vi "Remove Audio Files from NI ELVIS III.vi"() -> ()   [LabVIEW 2019]
doc: "This VI deletes all the Music files previously uploaded to the target. Only use this VI, after finishing using the Audio Modulation VIs or if you want to transfere other files."
uses:
  <vilib>/FTP/NI_FTP.lvlib
panel:
  in  "Message":string
  out "error out":errorcluster
  in  "error in (no error)":errorcluster
  in  "Host ID":string="172.22.11.2"
  # "Remove Audio Files from NI ELVIS III"
  # "This VI deletes all the Music files previously uploaded to the target. Only use this VI, after finishing using the Audio Modulation VIs or if you want to transfere other files.\n\nRemember that if you want to make use of the Demo once again, you should upload the Audio files once more to the NI ELVIS III."
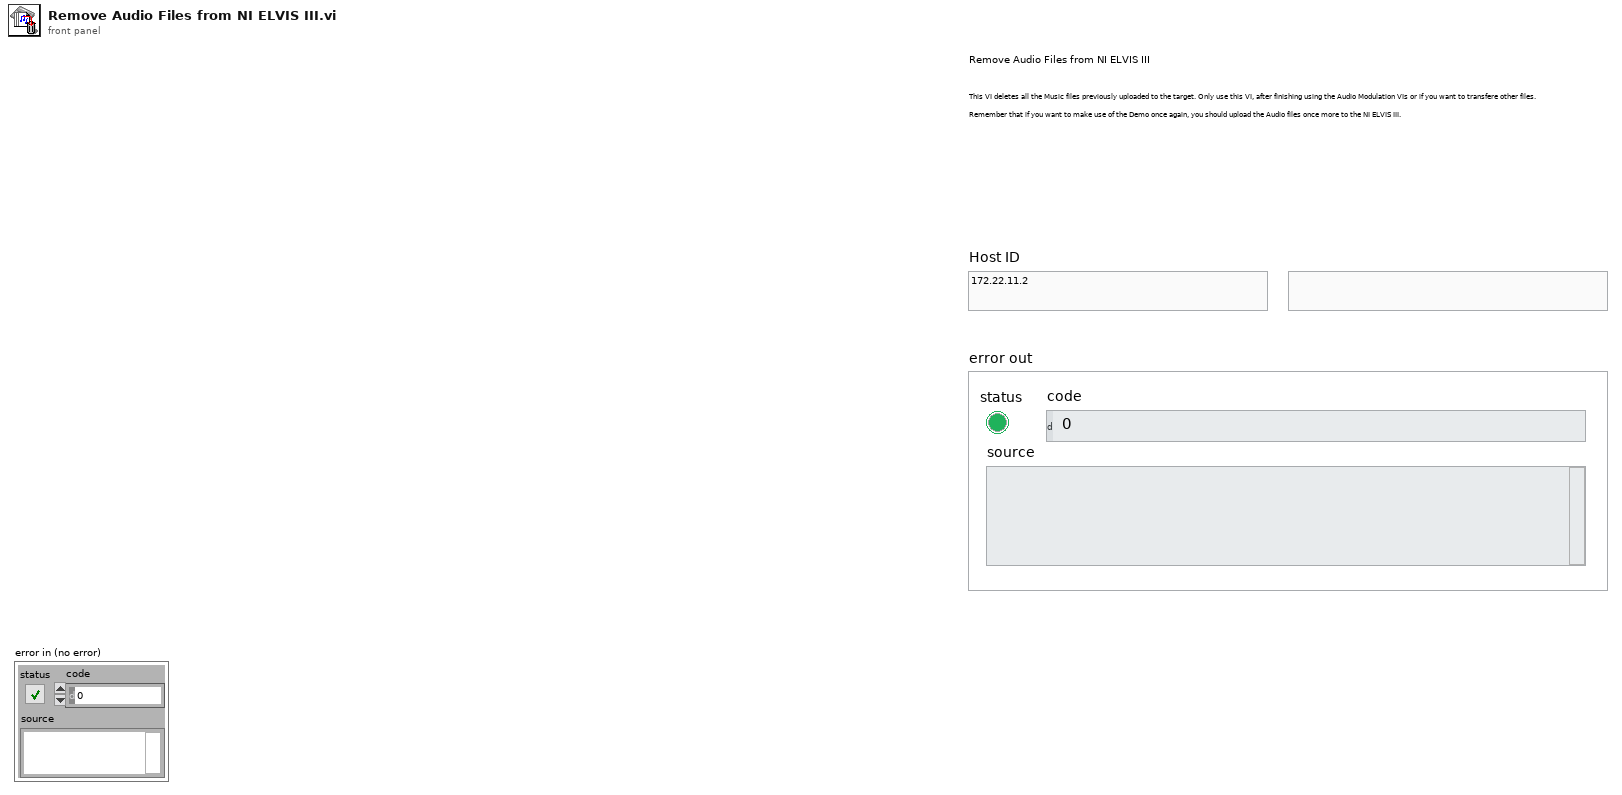
[diagram p1: front panel]
types:
  T1 = typedef "NI_FTP.lvlib/FTP Session.ctl" = refnum<k5>
  T2 = typedef "NI_FTP.lvlib/FTP File Info.ctl" = cluster{"type":enum16{"unknown", "file", "dir", "link"}, "permissions":string, "owner":string, "group":string, "size":i32, "date":string, "name":string, "link name":string}
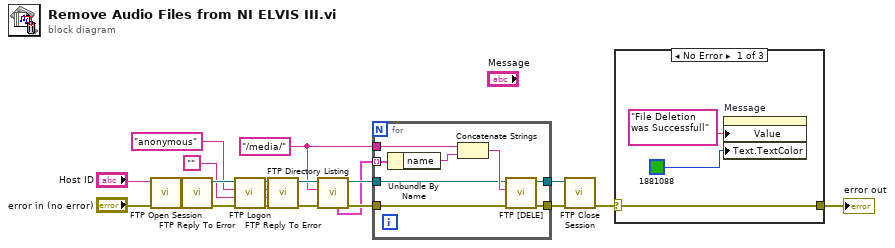
[diagram p0: block diagram]
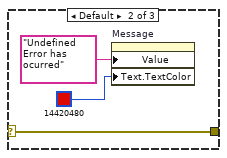
[diagram p2: hidden frame]
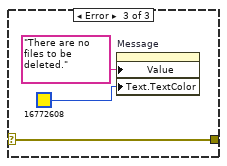
[diagram p3: hidden frame]
diagram:
  w4 = "/media/"
  n1 = call <vilib>:"FTP Open Session.vi"("error in (no error)"="error in (no error)", "address"="Host ID") -> ("error out"=w23:errorcluster, "reply string"=w21:string, "reply code"=w22:i32, "ftp session"=w24:T1)  [unwired: 2 in, 4 out]
  n2 = call <vilib>:"FTP Reply To Error.vi"("error in (no error)"=w23, "reply string in"=w21, "reply code in"=w22, "ftp session"=w24) -> ("error out"=w20:errorcluster, "ftp session out"=w19:T1)  [unwired: 2 out]
  n3 = call <vilib>:"FTP Logon.vi"("error in (no error)"=w20, "password"="", "user"="anonymous", "ftp session"=w19) -> ("error out"=w18:errorcluster, "reply string"=w16:string, "reply code"=w15:i32, "ftp session out"=w17:T1)  [unwired: 4 out]
  n4 = call <vilib>:"FTP Reply To Error.vi"("error in (no error)"=w18, "reply string in"=w16, "reply code in"=w15, "ftp session"=w17) -> ("error out"=w6:errorcluster, "ftp session out"=w5:T1)  [unwired: 2 out]
  n5 = call <vilib>:"FTP Directory Listing.vi"("error in (no error)"=w6, "directory path"=w4, "ftp session"=w5) -> ("error out"=w7:errorcluster, "ftp session out"=w8:T1, "dir list"=w3:T2[])  [unwired: 4 in, 2 out]
  n6 = for {
    tunnel: w4 -> [w27]
    tunnel: w8 -> [w29]
    tunnel: [w32] -> w14
    tunnel: w7 -> [w28]
    tunnel: [w31] -> w13
    tunnel: w3 -> [w26] mode=indexing
    n7 = Unbundle By Name(w26) -> ("name"=w25:string)
    n8 = Concatenate Strings(w27, w25) -> (w30:string)
    n9 = call <vilib>:"FTP [DELE].vi"("error in (no error)"=w28, "file path"=w30, "ftp session"=w29) -> ("error out"=w31:errorcluster, "ftp session out"=w32:T1)  [unwired: 5 in, 2 out]
  }
  n10 = call <vilib>:"FTP Close Session.vi"("error in (no error)"=w13, "ftp session"=w14) -> ("error out"=w2:errorcluster)  [unwired: 9 out]
  n11 = case shown="No Error" w2 {
    selector: w2 -> [w33 w36 w39]
    tunnel: [w33 w36 w39] -> w1
    frame No Error {
      n12 = property on="Message" class="Str"("Value"="File Deletion was Successfull" ("Message"), "Text.TextColor"=u32 1881088 ("Text.Text Colors:Text Color")) -> ()  [unwired: 2 in, 2 out]
    }
    frame Default {
      n13 = property on="Message" class="Str"("Value"="Undefined Error has ocurred" ("Message"), "Text.TextColor"=u32 14420480 ("Text.Text Colors:Text Color")) -> ()  [unwired: 2 in, 2 out]
    }
    frame Error {
      n14 = property on="Message" class="Str"("Value"="There are no files to be deleted." ("Message"), "Text.TextColor"=u32 16772608 ("Text.Text Colors:Text Color")) -> ()  [unwired: 2 in, 2 out]
    }
  }
  "error out" <- w1
